vi "GetSweepValues.vi"() -> ()   [LabVIEW 2010]
uses:
  <vilib>/addons/h5labview2/base/hid_t.ctl
  <vilib>/addons/h5labview2/dataset/H5Dread.llb/H5Dread.xnode
  <vilib>/addons/h5labview2/attrib/H5Aread.llb/H5Aread.xnode
  <vilib>/addons/h5labview2/base/lib_path.vi
  <vilib>/addons/h5labview2/base/H5Equery.vi
  <vilib>/addons/h5labview2/dataset/H5D.lvlib
  <vilib>/addons/h5labview2/space/H5S.lvlib
panel:
  out "Counter out":u64
  in  "sweep_list":string[](array[string])
  in  "Update size":i32=1000
  in  "Counter":i32
  in  "sweep_dim":u64[](array[numeric])
  in  "Sweep inst info":T1(array[cluster])=[{"Kind"=4, "Strings"=["3:7", "10.0.0.2", "V"], "uint64s"=[3, 7], "Doubles"=[0.30000001192092896, -2.0, 1.0, -1.0, 1.0], "DAQmx take out list"=[]}]
  in  "Exp File ref":T2 format="%.0x"
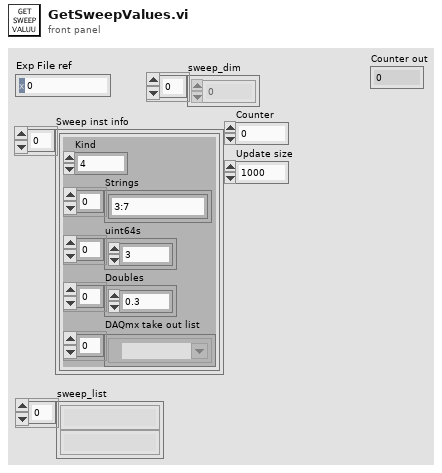
[diagram p1: front panel]
types:
  T1 = cluster{"Kind":u16, "Strings":string[], "uint64s":u64[], "Doubles":dbl[], "DAQmx take out list":refnum<k21>[]}[]
  T2 = typedef "hid_t.ctl" = i32
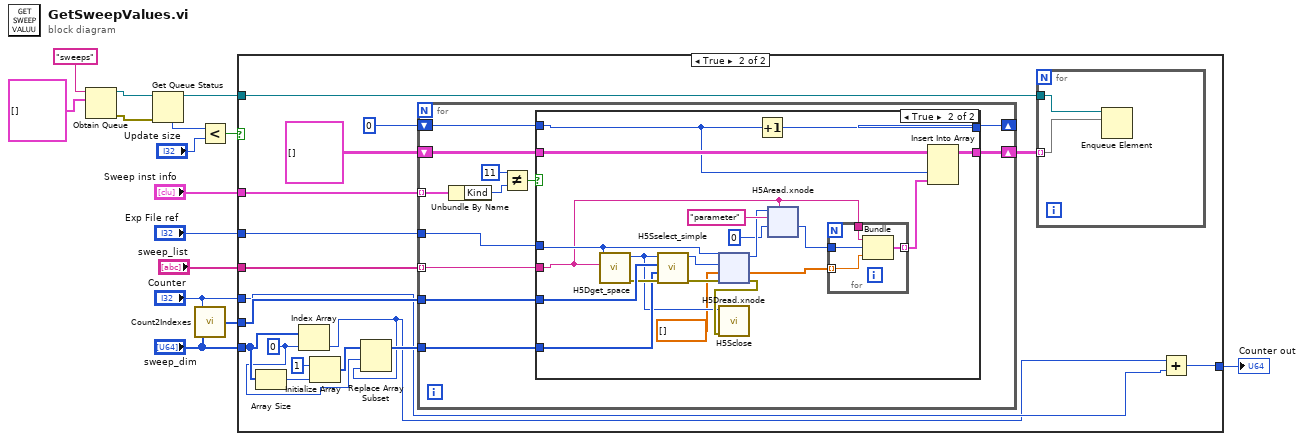
[diagram p0: block diagram]
diagram:
  n1 = Obtain Queue(name (unnamed)="sweeps", element data type=cluster{string, "data":u16, dbl}[] []) -> (queue out=w6:refnum<queue>, error out=w5:errorcluster)  [unwired: 3 in, 1 out]
  n2 = Get Queue Status(queue=w6, error in (no error)=w5) -> (queue out=w2:refnum<queue>, # elements in queue=w15:i32)  [unwired: 1 in, 6 out]
  n3 = call "Count2Indexes.vi"("sweep_dim"="sweep_dim", "Count"="Counter") -> ("Indexes"=w9:u64[])
  n4 = Less?(x=w15, y="Update size") -> (x < y?=w13:bool)
  n5 = case shown="True" w13 {
    tunnel: "Counter" -> [w16 w19]
    tunnel: "Exp File ref" -> [_ w27]
    tunnel: "Sweep inst info" -> [_ w28]
    tunnel: w9 -> [_ w25]
    tunnel: "sweep_dim" -> [_ w30]
    tunnel: "sweep_list" -> [_ w26]
    tunnel: w2 -> [_ w21]
    tunnel: [w16 w18] -> w1
    frame False {
    }
    frame True {
      w29 = 0
      n6 = Array Size(array=w30) -> (size(s)=w33:i32)
      n7 = Index Array(array=w30, index=w29) -> (element=w17:u64)
      n8 = Initialize Array(u32 1, w33) -> (w32:u32[])
      n9 = Replace Array Subset(array=w32, new element=w17, index=w29) -> (w24:u32[])
      n10 = for {
        tunnel: w28 -> [w47] mode=indexing
        tunnel: w27 -> [w42]
        tunnel: w26 -> [w43] mode=indexing
        tunnel: w25 -> [w41]
        tunnel: w24 -> [w40]
        shift-right: [w38] -> w20
        shift-left: cluster{string, "data":u16, dbl}[][] [] -> [w39]
        shift-right: [w36] -> _
        shift-left: u16 0 -> [w37]
        n11 = Unbundle By Name(w47) -> ("Kind"=w45:u16)
        n12 = Not Equal?(x=11, y=w45) -> (x != y?=w44:bool)
        n13 = case shown="True" w44 {
          tunnel: w43 -> [_ w53]
          tunnel: w42 -> [_ w65]
          tunnel: w41 -> [_ w69]
          tunnel: w40 -> [_ w67]
          tunnel: w39 -> [w49 w57]
          tunnel: [w49 w56] -> w38
          tunnel: w37 -> [w48 w50]
          tunnel: [w48 w55] -> w36
          frame False {
          }
          frame True {
            n14 = call <vilib>:"H5Dget_space.vi"("obj (.)"=w53, "ref in"=w65) -> ("error out"=w68:errorcluster, "space out"=w60:T2)  [unwired: 8 in]
            n15 = call <vilib>:"H5Sselect_simple.vi"("error in (no error)"=w68, "count"=w67, "start"=w69, "space in"=w60) -> ("error out"=w62:errorcluster, "space out"=w66:T2)  [unwired: 6 in]
            n16 = xnode "H5Dread.xnode"("error in (no error)"=w62, "default"=dbl[] [], "file space"=w66, "ref in"=w65) -> ("error out"=w61:errorcluster, "data"=w52:dbl[], "ref out"=w63:T2)  [unwired: 2 in, 1 out]
            n17 = call <vilib>:"H5Sclose.vi"("error in (no error)"=w61, "space in"=w60) -> ()  [unwired: 9 in, 1 out]
            n18 = Increment(x=w50) -> (x+1=w55:u16)
            n19 = xnode "H5Aread.xnode"("object name"=w53, "default"=u16 0, "attrib name"="parameter", "ref in"=w63) -> ("data"=w54:u16)  [unwired: 2 in, 3 out]
            n20 = for {
              tunnel: w54 -> [w73]
              tunnel: w53 -> [w72]
              tunnel: w52 -> [w71] mode=indexing
              tunnel: [w70] -> w51 mode=indexing
              n21 = Bundle(w72, "data"=w73, w71) -> (w70:cluster{string, "data":u16, dbl})  [unwired: 1 in]
            }
            n22 = Insert Into Array(array=w57, index (col)=w50, new element=w51) -> (w56:cluster{string, "data":u16, dbl}[][])  [unwired: 1 in]
          }
        }
      }
      n23 = for {
        tunnel: w21 -> [w35]
        tunnel: w20 -> [w34] mode=indexing
        n24 = Enqueue Element(queue=w35, element=w34) -> ()  [unwired: 2 in, 3 out]
      }
      n25 = Add(x=w17, y=w19) -> (x+y=w18:u64)
    }
  }
  "Counter out" <- w1
